vi "CloseExtendedSession.vi"(8 "error in (no error)":errorcluster, 11 "SessionID":string) -> (0 "error out":errorcluster)   [LabVIEW 2021, in "Lunar UDS CAN.lvlib"]
uses:
  Lunar UDS CAN.lvlib
  Controls/UDSActions.ctl
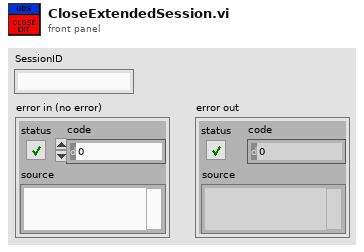
[diagram p1: front panel]
types:
  T1 = typedef "Lunar UDS CAN.lvlib/UDSActions.ctl" = enum16{"Open Session", "Connect To Diagnostic Session", "Send Tester Present", "ECU Reset", "Write String Data", "Write Byte Data", "Read Data", "Close Session", "Close All Sessions"}
  T2 = cluster{"Start Tester Present":bool, "Tester Present Period":dbl}
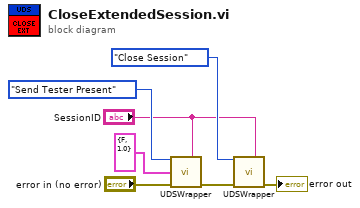
[diagram p0: block diagram]
diagram:
  n1 = call "UDSWrapper.vi"("UDS Action"=UDSActions."Send Tester Present", "SessionID"="SessionID", "Tester Present"=T2 {"Start Tester Present"=FALSE, "Tester Present Period"=1.0}, "error in (no error)"="error in (no error)") -> ("error out"=w5:errorcluster)  [unwired: 9 in, 2 out]
  n2 = call "UDSWrapper.vi"("UDS Action"=UDSActions."Close Session", "SessionID"="SessionID", "error in (no error)"=w5) -> ("error out"=→"error out":errorcluster)  [unwired: 10 in, 2 out]
